vi "Main.vi"() -> ()   [LabVIEW 2019]
doc: "The myRIO Project template acquires acceleration data from the onboard accelerometer and displays the changes of acceleration values in a waveform chart."
uses:
  <vilib>/myRIO/Common/Instrument Driver Framework/myRIO v1.0/Encoder/typedefs/Encoder Signal Mode.ctl
  <vilib>/myRIO/Instrument Drivers/Onboard IO/Encoder/typedefs/Encoder Reference.ctl
  <vilib>/myRIO/Common/Instrument Driver Framework/Utilities/typedefs/myRIO Generic Hardware Reference.ctl
  <vilib>/myRIO/Common/Instrument Driver Framework/Utilities/typedefs/Hardware Version Enum.ctl
  <vilib>/myRIO/Common/Instrument Driver Framework/Utilities/typedefs/myRIO v1.0 Reference.ctl
  <vilib>/myRIO/Common/Instrument Driver Framework/Utilities/typedefs/Generic FPGA Reference.ctl
  <vilib>/myRIO/Common/Instrument Driver Framework/myRIO v1.0/Encoder/typedefs/Encoder Channels Enum.ctl
  <vilib>/myRIO/Common/Instrument Driver Framework/myRIO v1.0/Encoder/typedefs/Encoder Configuration v1.0.ctl
  <vilib>/userdefined/High Color/nirio_resource_hc.ctl
  <vilib>/myRIO/Instrument Drivers/Onboard IO/DIO/typedefs/DIO Reference.ctl
  <vilib>/myRIO/Common/Instrument Driver Framework/myRIO v1.0/DIO/typedefs/DIO Channels List.ctl
  <vilib>/myRIO/Common/Instrument Driver Framework/myRIO v1.0/DIO/typedefs/DIO Channels Enum.ctl
  <vilib>/myRIO/Instrument Drivers/Onboard IO/AI/typedefs/AI Reference.ctl
  <vilib>/myRIO/Common/Instrument Driver Framework/myRIO v1.0/AI/typedefs/AI Channels List.ctl
  <vilib>/myRIO/Common/Instrument Driver Framework/myRIO v1.0/AI/typedefs/AI Channels Enum.ctl
  <vilib>/myRIO/Common/Instrument Driver Framework/Utilities/typedefs/Analog Scaling Constants List.ctl
  <vilib>/myRIO/Common/Instrument Driver Framework/Utilities/typedefs/Analog Scaling Constants.ctl
  <vilib>/myRIO/Instrument Drivers/Onboard IO/PWM/typedefs/PWM Reference.ctl
  <vilib>/myRIO/Common/Instrument Driver Framework/myRIO v1.0/PWM/typedefs/PWM Channels Enum.ctl
  <vilib>/myRIO/Instrument Drivers/Onboard IO/PWM/typedefs/PWM Configuration.ctl
  <vilib>/myRIO/Common/Instrument Driver Framework/Utilities/vis/Is FPGA Ref Available.vi
  <vilib>/myRIO/Common/Instrument Driver Framework/myRIO v1.0/Encoder/vis/myRIO v1.1 Open Encoder.vi
  <vilib>/myRIO/Instrument Drivers/Onboard IO/Encoder/vis/Read.vi
  <vilib>/myRIO/Common/Instrument Driver Framework/myRIO v1.0/AI/vis/myRIO v1.1 Open AI.vi
  <vilib>/myRIO/Instrument Drivers/Onboard IO/AI/vis/Read.vi
  <vilib>/myRIO/Common/Instrument Driver Framework/myRIO v1.0/DIO/vis/myRIO v1.1 Open DIO.vi
  <vilib>/myRIO/Instrument Drivers/Onboard IO/DIO/vis/Write.vi
  <vilib>/myRIO/Common/Instrument Driver Framework/myRIO v1.0/PWM/vis/myRIO v1.1 Open PWM.vi
  <vilib>/myRIO/Common/Instrument Driver Framework/Utilities/vis/Validate Channels.vi
  <vilib>/myRIO/Common/Instrument Driver Framework/myRIO v1.0/Encoder/vis/myRIO v1.0 Reserve Encoder.vi
  <vilib>/myRIO/Common/Instrument Driver Framework/myRIO v1.0/AI/vis/myRIO v1.0 Reserve AI.vi
  <vilib>/myRIO/Common/Instrument Driver Framework/myRIO v1.0/DIO/vis/myRIO v1.0 Reserve DIO.vi
  <vilib>/myRIO/Common/Instrument Driver Framework/myRIO v1.0/PWM/vis/myRIO v1.0 Reserve PWM.vi
  <vilib>/myRIO/Common/Instrument Driver Framework/myRIO v1.0/Encoder/vis/myRIO v1.0 Build MUX Configuration Encoder.vi
  <vilib>/myRIO/Common/Instrument Driver Framework/myRIO v1.0/Resource Manager/vis/myRIO v1.0 Reserve Channel List.vi
  <vilib>/myRIO/Common/Instrument Driver Framework/myRIO v1.0/AI/vis/myRIO v1.0 Build MUX Configuration AI.vi
  <vilib>/myRIO/Common/Instrument Driver Framework/myRIO v1.0/DIO/vis/myRIO v1.0 Build MUX Configuration DIO.vi
  <vilib>/myRIO/Common/Instrument Driver Framework/myRIO v1.0/PWM/vis/myRIO v1.0 Build MUX Configuration PWM.vi
  <vilib>/myRIO/Common/Instrument Driver Framework/myRIO v1.0/Resource Manager/vis/myRIO v1.0 Create Configuration List.vi
  <vilib>/myRIO/Common/Instrument Driver Framework/myRIO v1.0/Resource Manager/vis/myRIO v1.0 Reserve Channel.vi
  <vilib>/myRIO/Common/Instrument Driver Framework/myRIO v1.0/Resource Manager/vis/myRIO v1.0 Unreserve Channel.vi
  <vilib>/myRIO/Common/Instrument Driver Framework/myRIO v1.0/Resource Manager/vis/myRIO v1.0 Build Mutex Name.vi
  <vilib>/addons/control/pid/pid.llb/PID (DBL).vi
  <vilib>/Utility/VariantDataType/GetNumericInfo.vi
  <vilib>/Utility/error.llb/Error Cluster From Error Code.vi
  <vilib>/myRIO/Common/Instrument Driver Framework/myRIO v1.0/myRIO v1.1 Open.vi
  <vilib>/myRIO/Common/Instrument Driver Framework/Utilities/vis/IO Manager.vi
  <vilib>/myRIO/Common/Instrument Driver Framework/Utilities/vis/Configuration Manager.vi
  <vilib>/myRIO/Common/Instrument Driver Framework/myRIO v1.0/Resource Manager/vis/myRIO v1.0 Configure IO.vi
  <vilib>/myRIO/Common/Instrument Driver Framework/myRIO v1.0/myRIO v1.0 Close.vi
  <vilib>/myRIO/Common/Instrument Driver Framework/myRIO v1.0/Encoder/vis/myRIO v1.0 Configure Encoder.vi
  <vilib>/myRIO/Common/Instrument Driver Framework/myRIO v1.0/Encoder/vis/myRIO v1.0 Read Encoder.vi
  <vilib>/myRIO/Common/Instrument Driver Framework/myRIO v1.0/AI/vis/myRIO v1.0 Get Scaling Constants AI.vi
  <vilib>/myRIO/Common/Instrument Driver Framework/myRIO v1.0/AI/vis/myRIO v1.0 Read AI.vi
  <vilib>/myRIO/Common/Instrument Driver Framework/myRIO v1.0/PWM/vis/myRIO v1.0 Write PWM.vi
  <vilib>/myRIO/Common/Instrument Driver Framework/myRIO v1.0/DIO/vis/myRIO v1.0 Write DIO.vi
  <vilib>/myRIO/Express VI/Onboard IO/Encoder/Encoder Express VI.xnode
  <vilib>/myRIO/Common/Instrument Driver Framework/myRIO v1.0/Encoder/typedefs/Encoder Count Direction Enum.ctl
  <vilib>/myRIO/Instrument Drivers/Onboard IO/Encoder/vis/myRIO Encoder Open.xnode
  <vilib>/myRIO/Express VI/Onboard IO/AI/AI Express VI.xnode
  <vilib>/myRIO/Instrument Drivers/Onboard IO/AI/vis/myRIO AI Open.xnode
  <vilib>/myRIO/Express VI/Onboard IO/DO/DO Express VI.xnode
  <vilib>/myRIO/Instrument Drivers/Onboard IO/DIO/vis/myRIO DIO Open.xnode
  <vilib>/myRIO/Express VI/Onboard IO/PWM/PWM Express VI.xnode
  <vilib>/myRIO/Instrument Drivers/Onboard IO/PWM/vis/myRIO PWM Open.xnode
  <vilib>/myRIO/Instrument Drivers/Onboard IO/AI/AI.lvlib
  <vilib>/myRIO/Instrument Drivers/Onboard IO/Encoder/Encoder.lvlib
  <vilib>/myRIO/Instrument Drivers/Onboard IO/DIO/DIO.lvlib
  <vilib>/myRIO/Instrument Drivers/Onboard IO/PWM/PWM.lvlib
  <vilib>/addons/control/pid/NI_PID_pid.lvlib
panel:
  out "oFF2":dbl
  out "S1 2":dbl
  in  "Position 2":dbl
  out "Duty cycle 2":dbl
  out "Pulse Width 2 [ms]":dbl
  in  "stop":bool
  out "Frequency 2 [Hz] 3":dbl
  out "error out 5":errorcluster
  in  "error in (no error) 4":errorcluster
  out "rpm 2":i32
  in  "dirección 2":bool
  in  "Duty Cycle 2":dbl=0.5
  in  "dirección":bool
  in  "Duty Cycle":dbl=0.5
  out "Counter Direction 2":enum16{"Counting Up", "Counting Down"}(ring)
  out "rpm1":i32
  out "Counter Direction":enum16{"Counting Up", "Counting Down"}(ring)
  out "S4":dbl
  out "S3":dbl
  out "S2":dbl
  out "S1":dbl
  out "Boolean 4":bool
  out "Boolean 3":bool
  out "Boolean 2":bool
  out "Boolean":bool
  # "Overview: The myRIO Project template acquires acceleration data from the onboard accelerometer and displays the changes of acceleration values in a waveform chart.\nInstructions:\n1. Check the myRIO target IP address in the project and make sure the target IP address is correct. \n2. Run this VI."
  # "Motor 2"
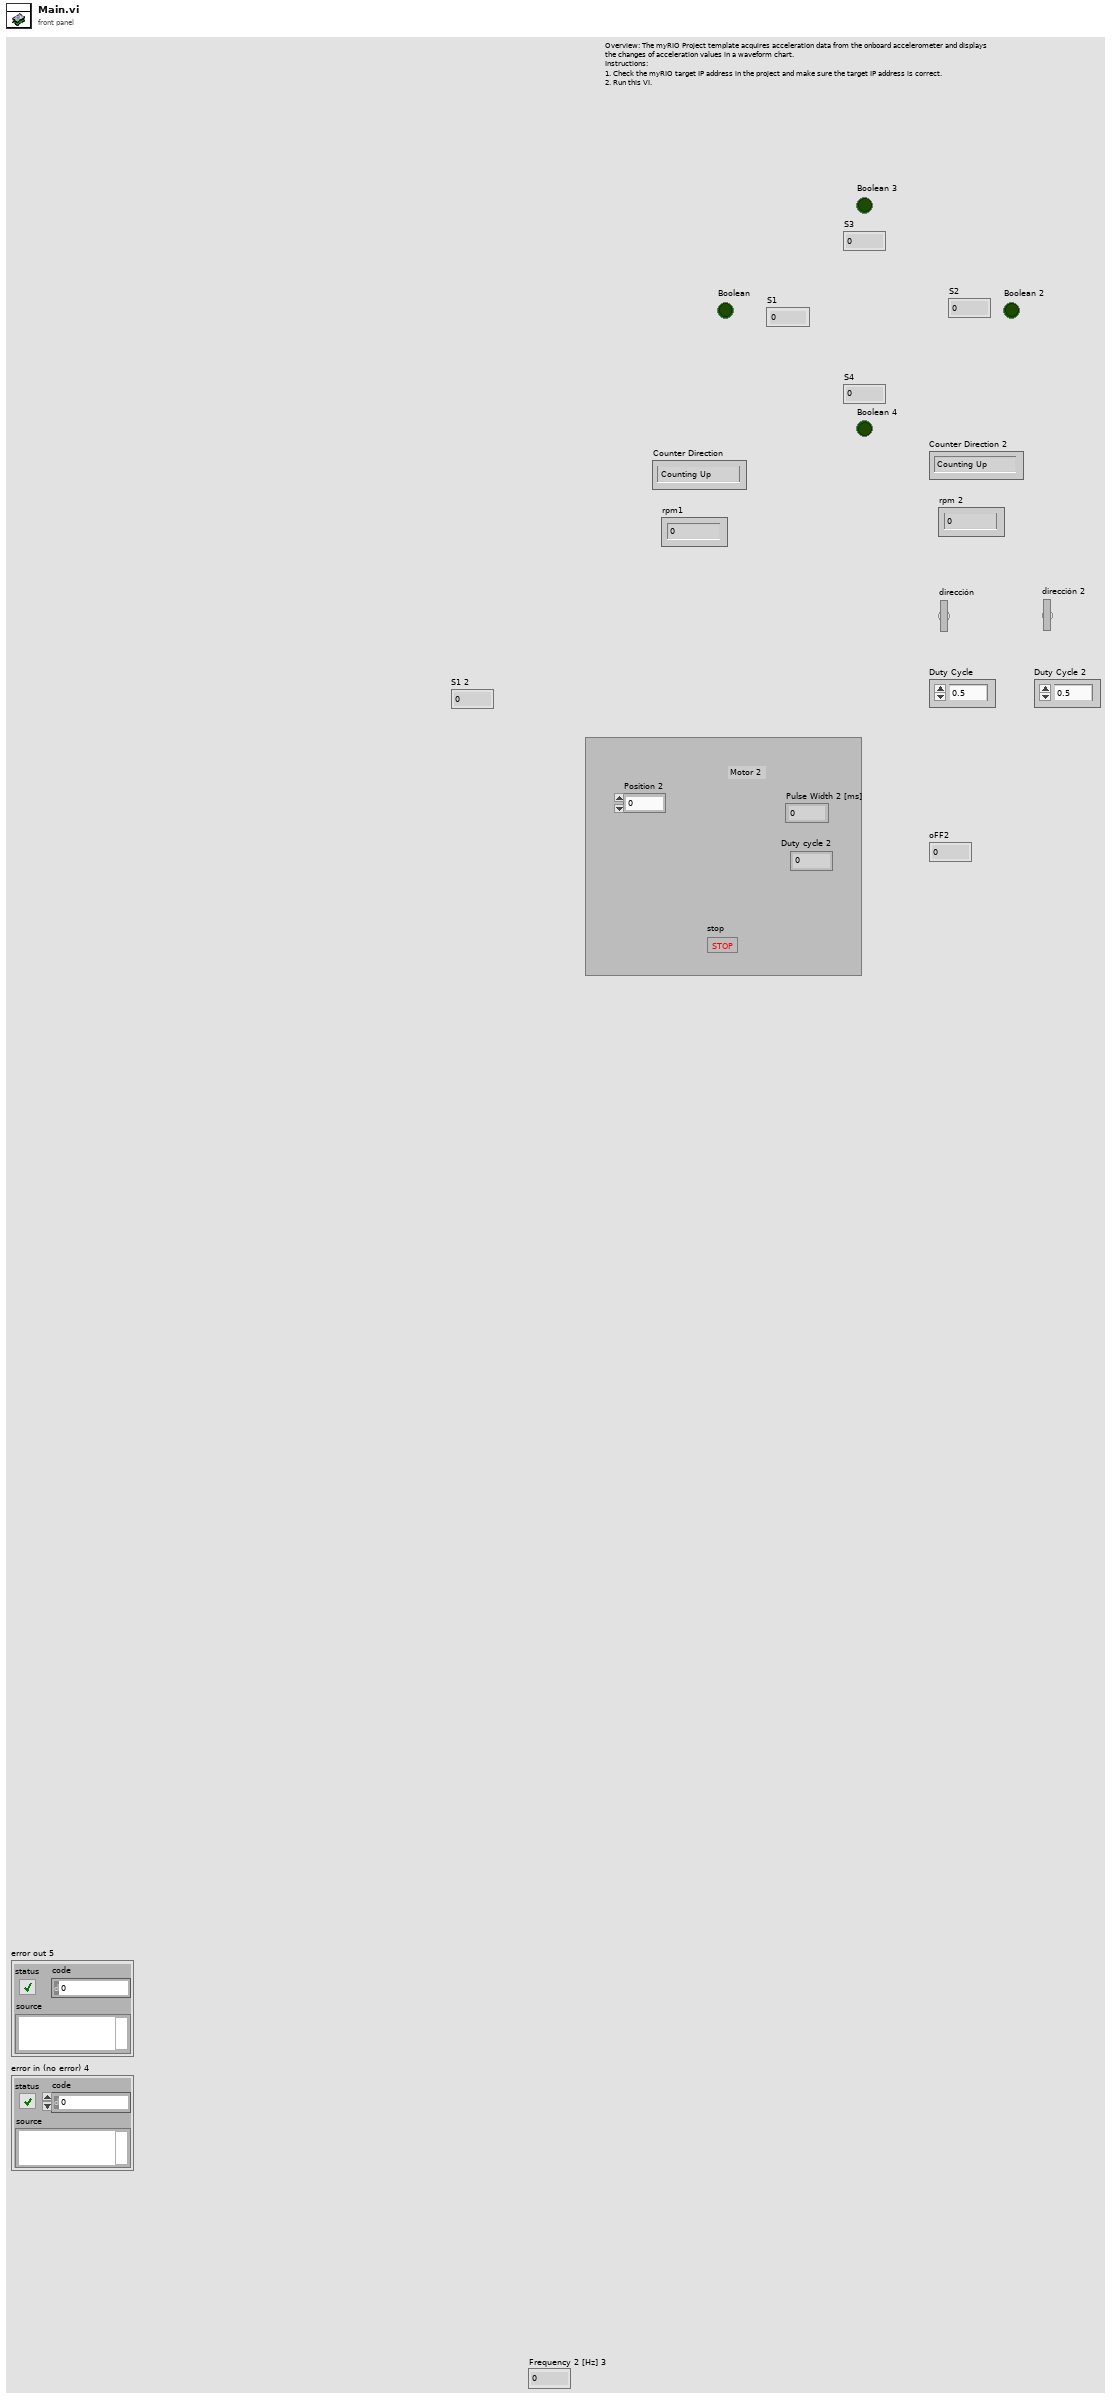
[diagram p1: front panel]
types:
  T1 = typedef "DIO.lvlib/DIO Reference.ctl" = cluster{"myRIO Reference":T2, "DIO Channels List":T6}
  T2 = typedef "myRIO Generic Hardware Reference.ctl" = cluster{"myRIO Model":T3, "myRIO Hardware Reference":T4}
  T3 = typedef "Hardware Version Enum.ctl" = enum16{"Unknown", "myRIO-1900", "myRIO-1950", "roboRIO", "NI ELVIS RIO CM", "ELVIS III"}
  T4 = typedef "myRIO v1.0 Reference.ctl" = cluster{"Generic FPGA Reference":T5, "Allow multiple opens":bool}
  T5 = typedef "Generic FPGA Reference.ctl" = refnum<k20>
  T6 = typedef "DIO Channels List.ctl" = T7[]
  T7 = typedef "DIO Channels Enum.ctl" = enum16{"Not Connected", "C/DIO0", "C/DIO1", "C/DIO2", "C/DIO3", "C/DIO4", "C/DIO5", "C/DIO6", "C/DIO7", "A/DIO0", "A/DIO1", "A/DIO2", "A/DIO3", "A/DIO4", "A/DIO5", "A/DIO6", "A/DIO7", "A/DIO8", "A/DIO9", "A/DIO10", "A/DIO11", "A/DIO12", "A/DIO13", "A/DIO14", "A/DIO15", "A/DIO16", "A/DIO17", "A/DIO18", "A/DIO19", "B/DIO0", "B/DIO1", "B/DIO2", "B/DIO3", "B/DIO4", "B/DIO5", "B/DIO6", "B/DIO7", "B/DIO8", "B/DIO9", "B/DIO10", "B/DIO11", "B/DIO12", "B/DIO13", "B/DIO14", "B/DIO15", "B/DIO16", "B/DIO17", "B/DIO18", "B/DIO19", "LED0", "LED1", "LED2", "LED3", "Button0", "DIO/DIO0", "DIO/DIO1", "DIO/DIO2", "DIO/DIO3", "DIO/DIO4", "DIO/DIO5", "DIO/DIO6", "DIO/DIO7", "DIO/DIO8", "DIO/DIO9", "SPI/CS0", "SPI/CS1", "SPI/CS2", "SPI/CS3", "LED RADIO (Green)", "LED RADIO (Red)", "LED COMM (Green)", "LED COMM (Red)", "LED MODE (Green)", "LED MODE (Red)"}
  T8 = typedef "nirio_resource_hc.ctl" = tag
  T9 = typedef "PWM.lvlib/PWM Reference.ctl" = cluster{"myRIO Reference":T2, "PWM Channels Enum":T10, "PWM Configuration":T11}
  T10 = typedef "PWM Channels Enum.ctl" = enum16{"Not Connected", "C/PWM0", "C/PWM1", "A/PWM0", "A/PWM1", "A/PWM2", "A/PWM3", "A/PWM4", "A/PWM5", "A/PWM6", "A/PWM7", "A/PWM8", "A/PWM9", "A/PWM10", "A/PWM11", "A/PWM12", "A/PWM13", "A/PWM14", "A/PWM15", "A/PWM16", "A/PWM17", "A/PWM18", "A/PWM19", "B/PWM0", "B/PWM1", "B/PWM2", "B/PWM3", "B/PWM4", "B/PWM5", "B/PWM6", "B/PWM7", "B/PWM8", "B/PWM9", "B/PWM10", "B/PWM11", "B/PWM12", "B/PWM13", "B/PWM14", "B/PWM15", "B/PWM16", "B/PWM17", "B/PWM18", "B/PWM19", "PWM/PWM0", "PWM/PWM1", "PWM/PWM2", "PWM/PWM3", "PWM/PWM4", "PWM/PWM5", "PWM/PWM6", "PWM/PWM7", "PWM/PWM8", "PWM/PWM9"}
  T11 = typedef "PWM.lvlib/PWM Configuration.ctl" = cluster{"Frequency":dbl, "Duty Cycle":dbl}
  T12 = typedef "Encoder.lvlib/Encoder Reference.ctl" = cluster{"myRIO Reference":T2, "Encoder Channels Enum":T13}
  T13 = typedef "Encoder Channels Enum.ctl" = enum16{"Not Connected", "C/ENC0", "C/ENC1", "A/ENC", "A/ENC0", "A/ENC1", "A/ENC2", "A/ENC3", "A/ENC4", "A/ENC5", "A/ENC6", "A/ENC7", "A/ENC8", "A/ENC9", "B/ENC", "B/ENC0", "B/ENC1", "B/ENC2", "B/ENC3", "B/ENC4", "B/ENC5", "B/ENC6", "B/ENC7", "B/ENC8", "B/ENC9", "DIO/ENC0", "DIO/ENC1", "DIO/ENC2", "DIO/ENC3", "DIO/ENC4"}
  T14 = typedef "Encoder Signal Mode.ctl" = enum16{"Quadrature phase signal", "Step and direction signal"}
  T15 = typedef "AI.lvlib/AI Reference.ctl" = cluster{"myRIO Reference":T2, "AI Channels List":T16, "AI Scaling Constants List":T18}
  T16 = typedef "AI Channels List.ctl" = T17[]
  T17 = typedef "AI Channels Enum.ctl" = enum16{"Not Connected", "AudioIn/Left", "AudioIn/Right", "C/AI0", "C/AI1", "A/AI0", "A/AI1", "A/AI2", "A/AI3", "A/AI4", "A/AI5", "A/AI6", "A/AI7", "B/AI0", "B/AI1", "B/AI2", "B/AI3", "B/AI4", "B/AI5", "B/AI6", "B/AI7", "AI/AI0", "AI/AI1", "AI/AI2", "AI/AI3", "A/AI0 (DIFF)", "A/AI1 (DIFF)", "A/AI2 (DIFF)", "A/AI3 (DIFF)", "B/AI0 (DIFF)", "B/AI1 (DIFF)", "B/AI2 (DIFF)", "B/AI3 (DIFF)"}
  T18 = typedef "Analog Scaling Constants List.ctl" = T19[]
  T19 = typedef "Analog Scaling Constants.ctl" = cluster{"LSB Weight (Volts)":dbl, "Offset (Volts)":dbl, "Signed?":bool}
  T20 = typedef "Encoder Count Direction Enum.ctl" = enum16{"Counting Up", "Counting Down"}
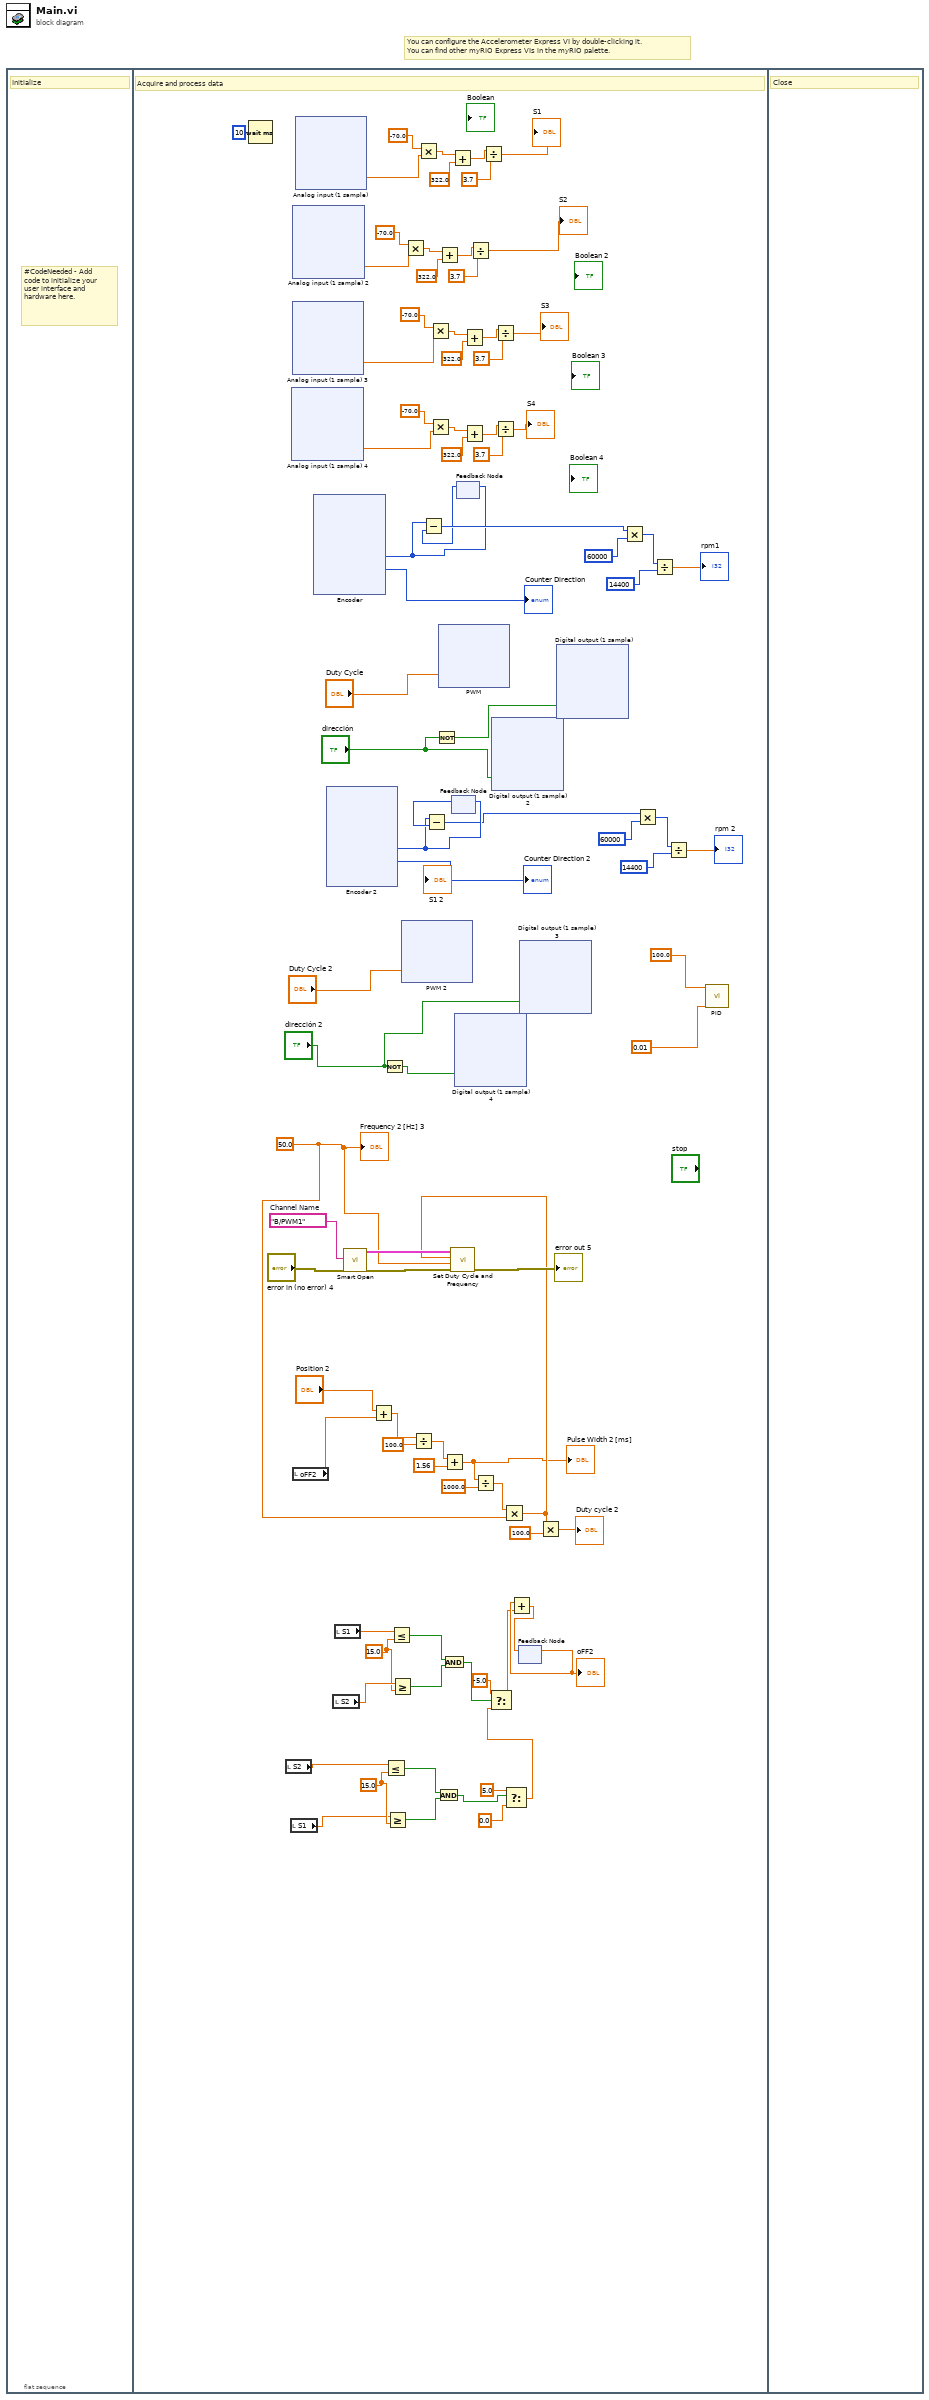
[diagram p0: block diagram]
diagram:
  # "You can configure the Accelerometer Express VI by double-clicking it.\nYou can find other myRIO Express VIs in the myRIO palette."
  n1 = flat-sequence {
    frame #0 {
      # "#CodeNeeded - Add code to initialize your user interface and hardware here."
      # "Initialize"
    }
    frame #1 {
      w9 = 15.0 ("y")
      w18 = 15.0 ("y")
      w24 = 50.0 ("Frequency 2 [Hz]")
      w32 = tag "B/PWM1"  # Channel Name
      # "Acquire and process data"
      n2 = Wait (ms)(milliseconds to wait=10) -> ()  [unwired: 1 out]
      n3 = local read "S2"() -> (w6:dbl)
      n4 = local read "S1"() -> (w5:dbl)
      n5 = xnode "Analog input (1 sample) 4"() -> ("A/AI3 (Pin 9)"=w65:dbl)  [unwired: 1 in, 1 out]
      n6 = xnode "Analog input (1 sample) 3"() -> ("A/AI2 (Pin 7)"=w78:dbl)  [unwired: 1 in, 1 out]
      n7 = local read "oFF2"() -> (w15:dbl)
      n8 = xnode "Analog input (1 sample) 2"() -> ("A/AI1 (Pin 5)"=w90:dbl)  [unwired: 1 in, 1 out]
      n9 = xnode "Analog input (1 sample)"() -> ("A/AI0 (Pin 3)"=w71:dbl)  [unwired: 1 in, 1 out]
      n10 = xnode "Encoder"() -> ("Counter Value"=w47:i32, "Counter Direction"=→"Counter Direction":enum16{"Counting Up", "Counting Down"})  [unwired: 2 in, 2 out]
      n11 = xnode "Encoder 2"() -> ("Counter Value"=w39:i32, "Counter Direction"=→"Counter Direction 2":T20)  [unwired: 2 in, 2 out]
      n12 = local read "S2"() -> (w19:dbl)
      n13 = local read "S1"() -> (w20:dbl)
      n14 = call <vilib>:"Smart Open.vi"("error in (no error)"="error in (no error) 4", "Channel Name"=w32) -> ("error out"=w29:errorcluster, "PWM Ref Out"=w30:T9)  [unwired: 8 in]
      n15 = Add(x="Position 2", y=w15) -> (x+y=w36:dbl)
      n16 = Not(x="dirección 2") -> (.not. x?=w57:bool)
      n17 = Less Or Equal?(x=w6, y=w9) -> (x <= y?=w8:bool)
      n18 = Greater Or Equal?(x=w5, y=w9) -> (x >= y?=w7:bool)
      n19 = Less Or Equal?(x=w20, y=w18) -> (x <= y?=w17:bool)
      n20 = Greater Or Equal?(x=w19, y=w18) -> (x >= y?=w16:bool)
      n21 = xnode "PWM 2"("Duty Cycle"="Duty Cycle 2") -> ()  [unwired: 1 in, 1 out]
      n22 = Multiply(x=-70.0, y=w90) -> (x*y=w88:dbl)
      n23 = Divide(x=w36, y=100.0) -> (x/y=w37:dbl)
      n24 = Multiply(x=-70.0, y=w71) -> (x*y=w75:dbl)
      n25 = Multiply(x=-70.0, y=w78) -> (x*y=w82:dbl)
      n26 = Multiply(x=-70.0, y=w65) -> (x*y=w68:dbl)
      n27 = Not(x="dirección") -> (.not. x?=w60:bool)
      n28 = And(x=w8, y=w7) -> (x .and. y?=w3:bool)
      n29 = Add(x=w88, y=322.0) -> (x+y=w85:dbl)
      n30 = xnode "PWM"("Duty Cycle"="Duty Cycle") -> ()  [unwired: 1 in, 1 out]
      n31 = Add(x=w37, y=1.56) -> (x+y=w22:dbl)
      "Pulse Width 2 [ms]" <- w22
      n32 = And(x=w17, y=w16) -> (x .and. y?=w12:bool)
      n33 = Add(x=w75, y=322.0) -> (x+y=w73:dbl)
      n34 = feedback #1() -> (w44:i32)  [unwired: 1 in]
      n35 = Subtract(x=w39, y=w44) -> (x-y=w38:i32)
      n36 = feedback-in #1(w39) -> ()
      n37 = xnode "Digital output (1 sample) 4"("B/DIO10 (Pin 31)"=w57) -> ()  [unwired: 1 in, 1 out]
      n38 = feedback-in #2(w47) -> ()
      n39 = feedback #2() -> (w45:i32)  [unwired: 1 in]
      n40 = Subtract(x=w47, y=w45) -> (x-y=w49:i32)
      n41 = Add(x=w82, y=322.0) -> (x+y=w80:dbl)
      n42 = Add(x=w68, y=322.0) -> (x+y=w66:dbl)
      n43 = Divide(x=w85, y=3.7 ("x")) -> (x/y=→"S2":dbl)
      n44 = Divide(x=w22, y=1000.0) -> (x/y=w27:dbl)
      n45 = Divide(x=w73, y=3.7 ("x")) -> (x/y=→"S1":dbl)
      n46 = xnode "Digital output (1 sample) 2"("A/DIO7 (Pin 25)"="dirección") -> ()  [unwired: 1 in, 1 out]
      n47 = Divide(x=w80, y=3.7 ("x")) -> (x/y=→"S3":dbl)
      n48 = Divide(x=w66, y=3.7 ("x")) -> (x/y=→"S4":dbl)
      n49 = Multiply(x=w27, y=w24) -> (x*y=w25:dbl)
      n50 = call <vilib>:"Set Duty Cycle and Frequency.vi"("error in (no error)"=w29, "Frequency [Hz]"=w24, "Duty Cycle"=w25, "PWM Ref In"=w30) -> ("error out"=→"error out 5":errorcluster)  [unwired: 5 in, 1 out]
      n51 = Select(t=5.0, s=w3, f=0.0) -> (s? t:f=w1:dbl)
      n52 = Select(t=-5.0, s=w12, f=w1) -> (s? t:f=w10:dbl)
      n53 = feedback #3() -> (w13:dbl)  [unwired: 1 in]
      "oFF2" <- w13
      n54 = Add(x=w13, y=w10) -> (x+y=w14:dbl)
      n55 = feedback-in #3(w14) -> ()
      n56 = xnode "Digital output (1 sample) 3"("B/DIO7 (Pin 25)"="dirección 2") -> ()  [unwired: 1 in, 1 out]
      n57 = Multiply(x=w25, y=100.0) -> (x*y=→"Duty cycle 2":dbl)
      n58 = xnode "Digital output (1 sample)"("A/DIO10 (Pin 31)"=w60) -> ()  [unwired: 1 in, 1 out]
      n59 = Multiply(x=w49, y=60000) -> (x*y=w48:i32)
      n60 = Multiply(x=w38, y=60000) -> (x*y=w41:i32)
      n61 = Divide(x=w48, y=14400) -> (x/y=→"rpm1":dbl)
      n62 = Divide(x=w41, y=14400) -> (x/y=→"rpm 2":dbl)
      n63 = call-poly <vilib>:"PID.vi"("dt (s)"=0.01, "setpoint"=100.0) -> ()  [unwired: 8 in, 2 out]
      "Frequency 2 [Hz] 3" <- w24
    }
    frame #2 {
      # "Close"
    }
  }
